vi "NetVarWrite_dbl.vi"(10 "Numeric":dbl, 11 "Refnum in":refnum<k21>) -> ()   [LabVIEW 2016, in "IPS-120.lvlib"]
uses:
  IPS-120.lvlib
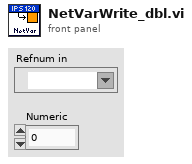
[diagram p1: front panel]
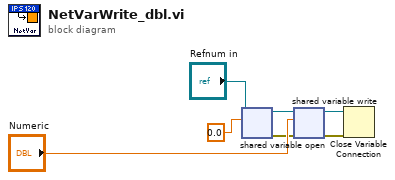
[diagram p0: block diagram]
diagram:
  n1 = shared-variable-open("Refnum in", 0.0) -> (w3:refnum<k21>, w2:errorcluster)  [unwired: 2 in]
  n2 = shared-variable-write(w3, w2, "Numeric") -> (w4:refnum<k21>, w1:errorcluster)
  n3 = Close Variable Connection(8:w1, 11:w4) -> ()  [unwired: 1 out]
